vi "UTIL_ATPStatus.vi"(8 "ChB!ChA":bool, 9 "Drain!Fill":bool, 10 "Status In in":i16, 11 "Good!Bad":bool) -> (1 "Err Num":u32, 2 "Bad Switch":bool, 3 "Status In out":u32)   [LabVIEW 2024]
uses:
  Control Definitions/Def_ATPStatus.ctl
panel:
  in  "Error Rng OK":bool
  out "Status":T1
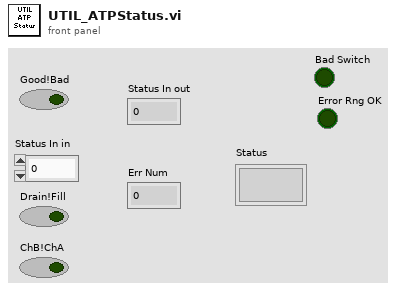
[diagram p1: front panel]
types:
  T1 = typedef "Def_ATPStatus.ctl" = i16
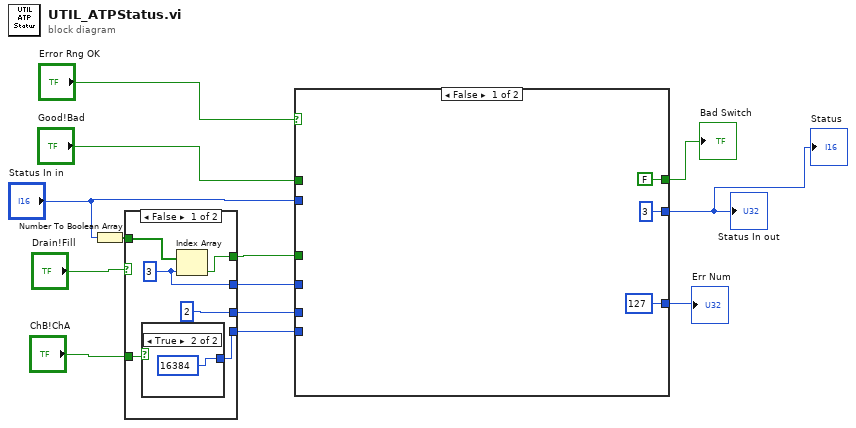
[diagram p0: block diagram]
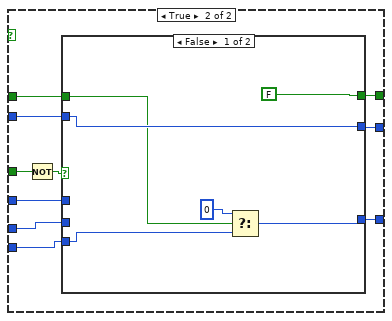
[diagram p2: hidden frame]
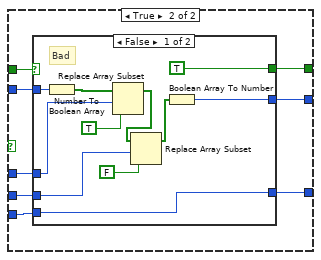
[diagram p3: hidden frame]
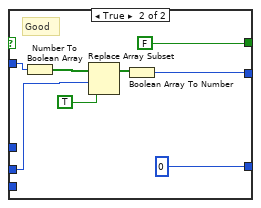
[diagram p4: hidden frame]
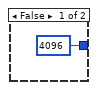
[diagram p5: hidden frame]
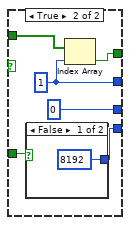
[diagram p6: hidden frame]
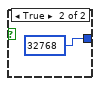
[diagram p7: hidden frame]
diagram:
  n1 = Number To Boolean Array(number="Status In in") -> (Boolean array=w8:bool[])
  n2 = case shown="False" "Drain!Fill" {
    tunnel: w8 -> [w19 w26]
    tunnel: [w18 w27] -> w7
    tunnel: [2 ("index") 0 ("index")] -> w6
    tunnel: [w16 w24] -> w5
    tunnel: [w15 w23] -> w3
    tunnel: "ChB!ChA" -> [w14 w22]
    frame False {
      w16 = 3 ("index")
      n3 = case shown="True" w14 {
        tunnel: [4096 ("index") 16384 ("index")] -> w15
        frame False {
        }
        frame True {
        }
      }
      n4 = Index Array(array=w19, index=w16) -> (element=w18:bool)
    }
    frame True {
      w24 = 1 ("index")
      n5 = case shown="False" w22 {
        tunnel: [8192 ("index") 32768 ("index")] -> w23
        frame False {
        }
        frame True {
        }
      }
      n6 = Index Array(array=w26, index=w24) -> (element=w27:bool)
    }
  }
  n7 = case shown="False" "Error Rng OK" {
    tunnel: "Status In in" -> [_ w42]
    tunnel: "Good!Bad" -> [_ w40]
    tunnel: [u32 127 ("Err Num") w39] -> w11
    tunnel: [FALSE w38] -> w10
    tunnel: w7 -> [_ w37]
    tunnel: w6 -> [_ w36]
    tunnel: w5 -> [_ w35]
    tunnel: [u32 3 ("Status In in") w34] -> w4
    tunnel: w3 -> [_ w33]
    frame False {
    }
    frame True {
      n8 = Not(x=w37) -> (.not. x?=w41:bool)
      n9 = case shown="False" w41 {
        tunnel: w40 -> [w46 w56]
        tunnel: [w48 w55] -> w34
        tunnel: w42 -> [w48 w54]
        tunnel: [w47 w53] -> w39
        tunnel: [FALSE w52] -> w38
        tunnel: w36 -> [_ w51]
        tunnel: w35 -> [_ w50]
        tunnel: w33 -> [w43 w49]
        frame False {
          n10 = Select(t=0, s=w46, f=w43) -> (s? t:f=w47:i32)
        }
        frame True {
          n11 = case shown="False" w56 {
            tunnel: w54 -> [w66 w74]
            tunnel: [w64 w71] -> w55
            tunnel: [w57 u32 0 ("Err Num")] -> w53
            tunnel: [TRUE FALSE] -> w52
            tunnel: w51 -> [w58 w68]
            tunnel: w50 -> [w59 _]
            tunnel: w49 -> [w57 _]
            frame False {
              # "Bad"
              n12 = Number To Boolean Array(number=w66) -> (Boolean array=w65:bool[])
              n13 = Replace Array Subset(array=w65, new element=TRUE ("new element/subarray"), index=w59) -> (w62:bool[])
              n14 = Replace Array Subset(array=w62, new element=FALSE ("new element/subarray"), index=w58) -> (w61:bool[])
              n15 = Boolean Array To Number(Boolean array=w61) -> (number=w64:u32)
            }
            frame True {
              # "Good"
              n16 = Number To Boolean Array(number=w74) -> (Boolean array=w73:bool[])
              n17 = Replace Array Subset(array=w73, new element=TRUE ("new element/subarray"), index=w68) -> (w72:bool[])
              n18 = Boolean Array To Number(Boolean array=w72) -> (number=w71:u32)
            }
          }
        }
      }
    }
  }
  "Status In out" <- w4
  "Err Num" <- w11
  "Bad Switch" <- w10
  "Status" <- w4
